vi "Read Sub Panel Prod.vi"(8 "error in (no error)":errorcluster, 11 "Doña Rata Actor in":refnum<class "Doña Rata Actor.lvclass">) -> (0 "error out":errorcluster, 2 "Sub Panel Prod":refnum<vi>, 3 "Doña Rata Actor out":refnum<class "Doña Rata Actor.lvclass">)   [LabVIEW 2020, in "Doña Rata Actor.lvlib" / "Doña Rata Actor.lvclass"]
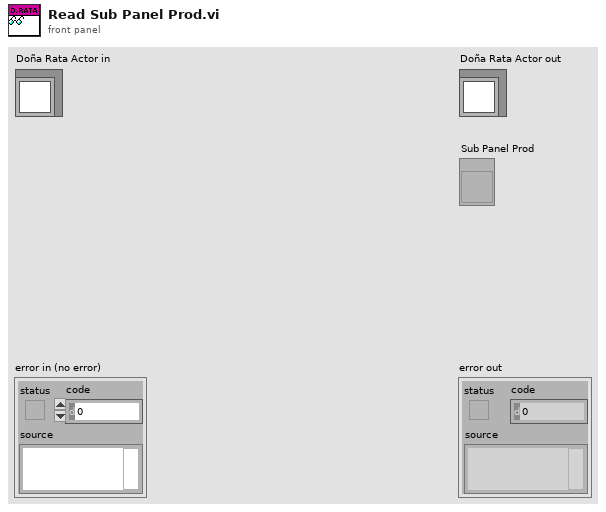
[diagram p1: front panel]
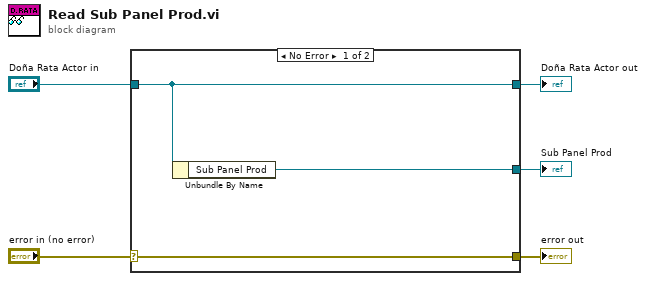
[diagram p0: block diagram]
diagram:
  n1 = case shown="No Error" "error in (no error)" {
    selector: "error in (no error)" -> [w8 w9]
    tunnel: [w8 w9] -> w4
    tunnel: [w7 w10] -> w2
    tunnel: "Doña Rata Actor in" -> [w7 w10]
    tunnel: [w6 _] -> w1
    frame No Error {
      n2 = Unbundle By Name(w7) -> ("Sub Panel Prod"=w6:refnum<vi>)
    }
    frame Error {
    }
  }
  "error out" <- w4
  "Doña Rata Actor out" <- w2
  "Sub Panel Prod" <- w1
